vi "practica2_ejercicio2i.vi"() -> ()   [LabVIEW 2011]
panel:
  in  "stop":bool
  in  "RETARDO":dbl(slide) scale=0.0..10.0
  in  "FRECUENCIA 2":dbl(slide) scale=0.0..10.0
  in  "FRECUENCIA":dbl(slide) scale=0.0..10.0
  out "Waveform Chart":dynamicdata(graph)
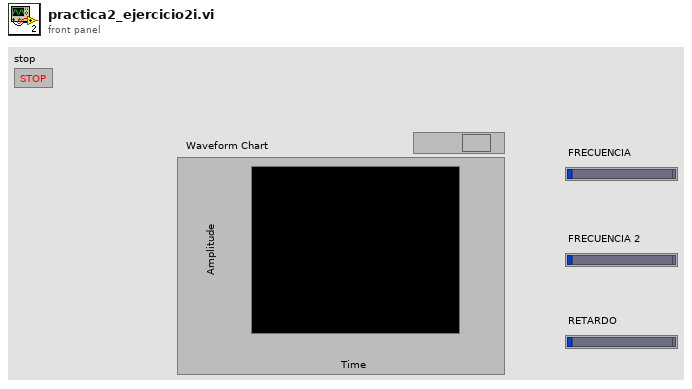
[diagram p1: front panel]
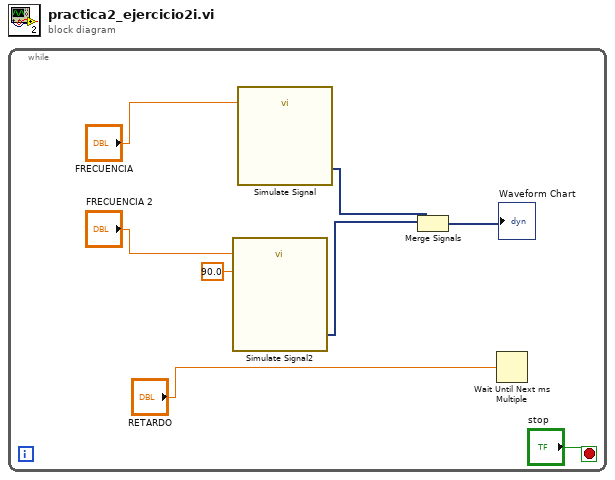
[diagram p0: block diagram]
diagram:
  n1 = while {
    stop <- "stop" stop-if-true
    n2 = call "Simulate Signal2"("Frequency"="FRECUENCIA 2", "Phase"=90.0) -> ("Sine"=w5:dynamicdata)  [unwired: 12 in, 1 out]
    n3 = call "Simulate Signal"("Frequency"="FRECUENCIA") -> ("Sine"=w6:dynamicdata)  [unwired: 13 in, 1 out]
    n4 = Merge Signals(w6, w5) -> (→"Waveform Chart":dynamicdata)
    n5 = Wait Until Next ms Multiple(millisecond multiple="RETARDO") -> ()  [unwired: 1 out]
  }
